vi "setArduinoMicro.vi"(5 "Enable":bool=TRUE, 8 "error in":errorcluster, 9 "ESTADO":T1, 11 "VISA resource name":refnum<visa-resource-name>="COM25") -> (0 "error out":errorcluster, 1 "ESTADO 2":T1)   [LabVIEW 2017]
uses:
  KISSIA_VALVULAS.ctl
  ArduinoMicro Module Control.ctl
panel:
  out "ERROR":bool
  out "write string":string
  out "read string":string
  out "TIMEOUT":bool
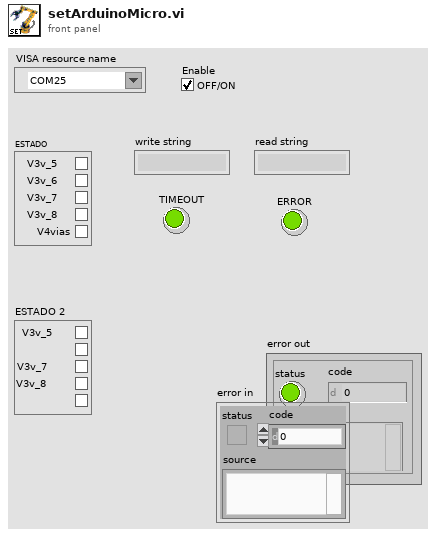
[diagram p1: front panel]
types:
  T1 = typedef "KISSIA_VALVULAS.ctl" = cluster{"V3v_5":bool, "V3v_6":bool, "V3v_7":bool, "V3v_8":bool, "V4vias":bool}
  T2 = typedef "ArduinoMicro Module Control.ctl" = enum16{"Initialize", "Read Data", "Write Data", "Enable", "Disable", "Shutdown"}
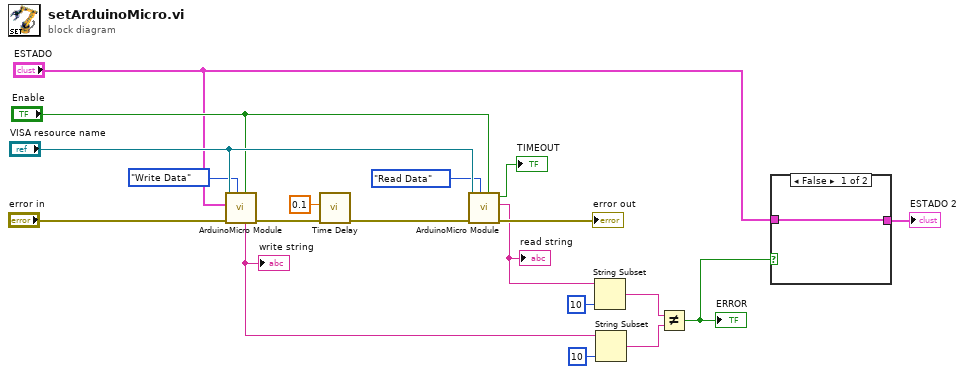
[diagram p0: block diagram]
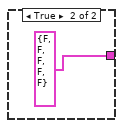
[diagram p2: hidden frame]
diagram:
  n1 = call "ArduinoMicro Module.vi"("Enable"="Enable", "Command"=ArduinoMicro_Module_Control."Write Data", "error in (no error)"="error in", "VALVES"="ESTADO", "VISA resource name"="VISA resource name") -> ("error out"=w11:errorcluster, "write string"=w8:string)  [unwired: 2 in, 3 out]
  "write string" <- w8
  n2 = call "Time Delay"("error in (no error)"=w11, "Delay Time (s)"=0.1) -> ("error out"=w10:errorcluster)  [unwired: 9 in]
  n3 = call "ArduinoMicro Module.vi"("Enable"="Enable", "Command"=ArduinoMicro_Module_Control."Read Data", "error in (no error)"=w10, "VISA resource name"="VISA resource name") -> ("error out"=→"error out":errorcluster, "read string"=w6:string, "TimeOut"=→"TIMEOUT":bool)  [unwired: 3 in, 2 out]
  "read string" <- w6
  n4 = String Subset(string=w6, length (rest)=10 ("length (rest)")) -> (substring=w5:string)  [unwired: 1 in]
  n5 = String Subset(string=w8, length (rest)=10 ("length (rest)")) -> (substring=w4:string)  [unwired: 1 in]
  n6 = Not Equal?(x=w5, y=w4) -> (x != y?=w3:bool)
  "ERROR" <- w3
  n7 = case shown="False" w3 {
    tunnel: "ESTADO" -> [w20 _]
    tunnel: [w20 T1 {"V3v_5"=FALSE, "V3v_6"=FALSE, "V3v_7"=FALSE, "V3v_8"=FALSE, "V4vias"=FALSE} ("ESTADO 2")] -> w1
    frame False {
    }
    frame True {
    }
  }
  "ESTADO 2" <- w1
